vi "Commascript advanced.vi"() -> ()   [LabVIEW 2017]
panel:
  out "concatenated string":string
  out "stripped path":path
  out "appended path":path
  out "stripped path 2":path
  in  "Starting Pos":i16(slide)=128 scale=340.0..50.0
  in  "string":string
  out "new picture":picture
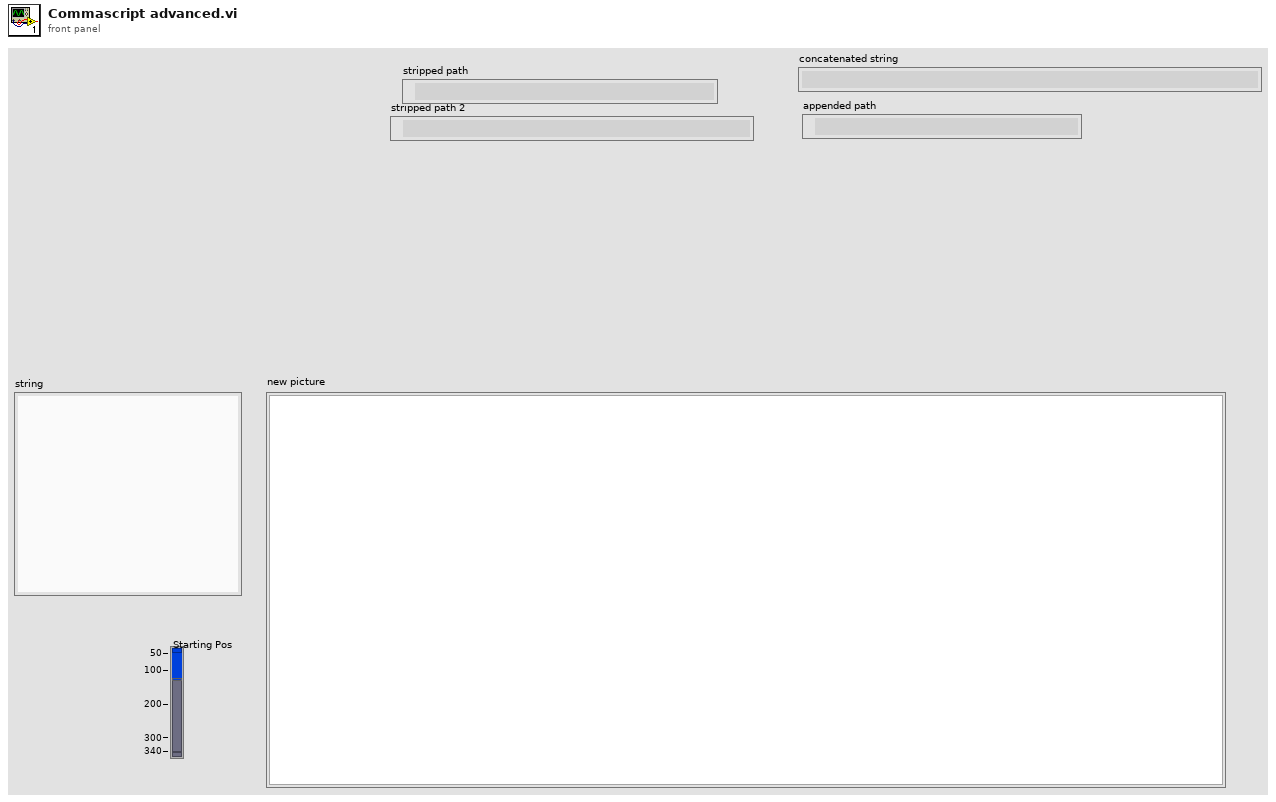
[diagram p1: front panel]
types:
  T1 = enum32{"invalid app kind", "Development System", "Run Time System", "Student Edition", "Embedded LabVIEW", "Evaluation", "Custom"}
  T2 = typedef "imagedata.ctl" = cluster{"image type":i32, "image depth":i32, "image":u8[], "mask":u8[], "colors":u32[], "Rectangle":cluster{"left":i16, "top":i16, "right":i16, "bottom":i16}}
  T3 = cluster{"Width":u16, "Style":enum32{"Solid", "Dash", "Dot", "DashDot", "DashDotDot"}}
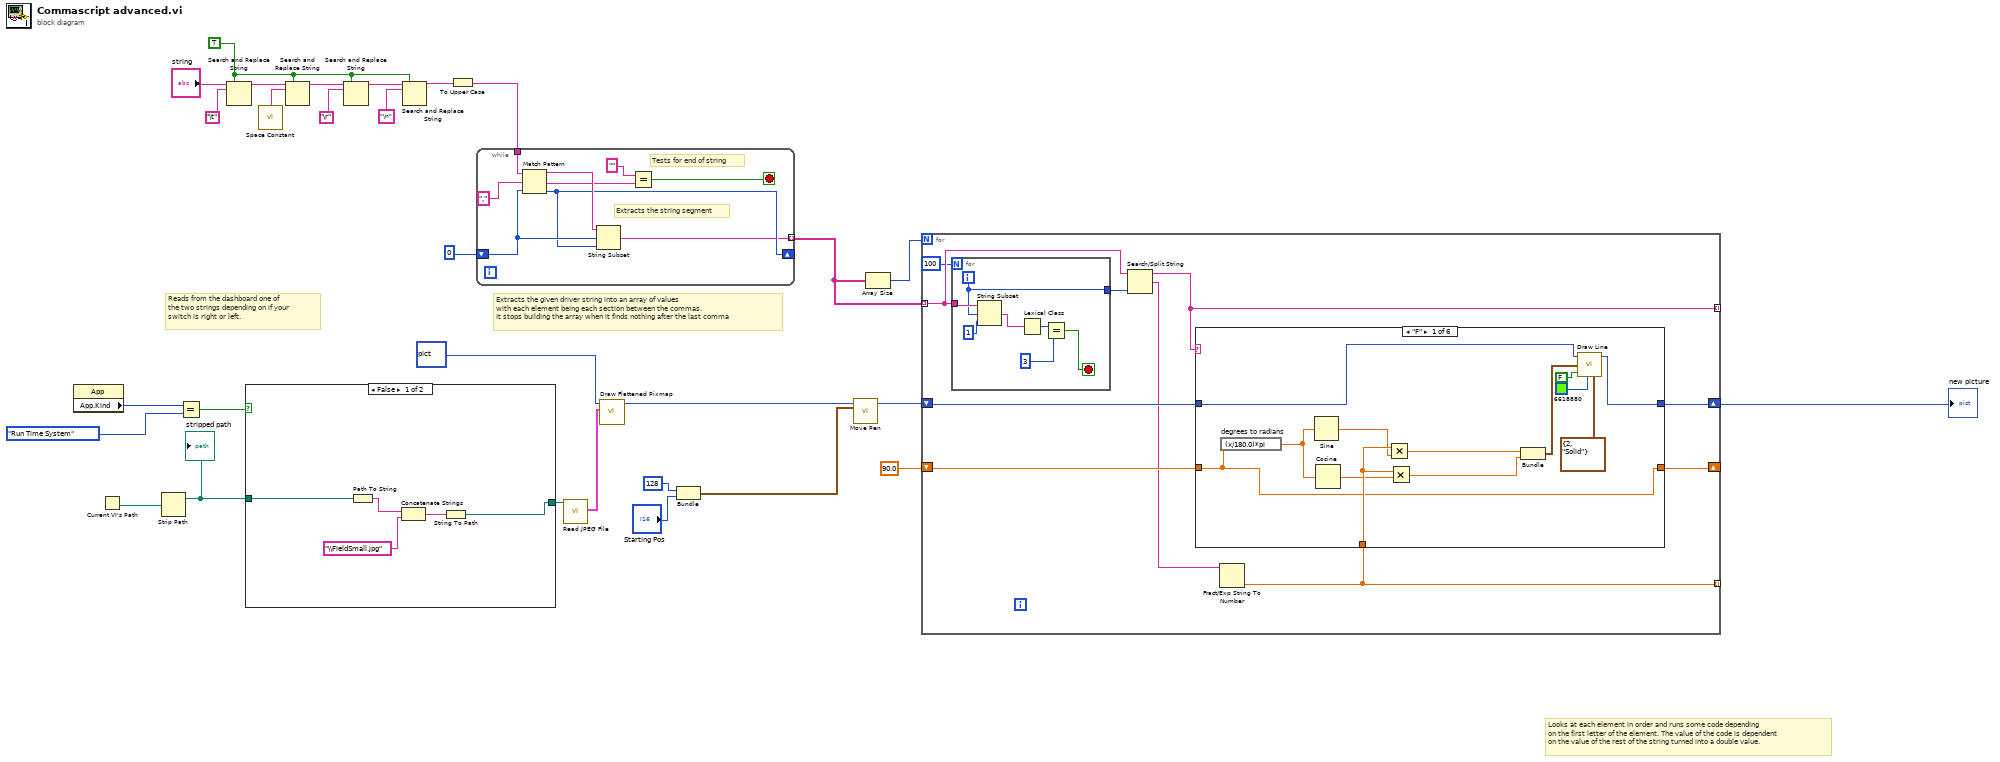
[diagram p0: block diagram]
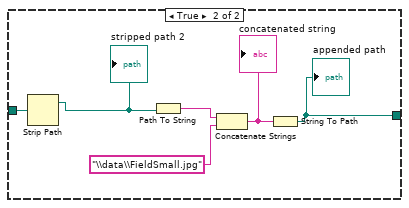
[diagram p2: hidden frame]
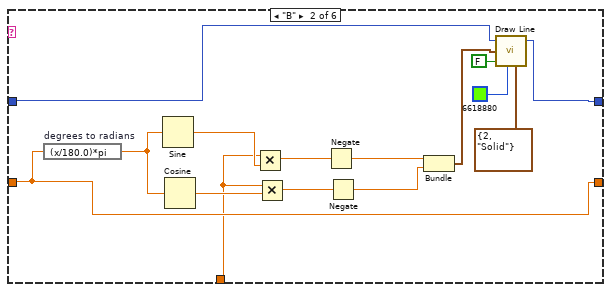
[diagram p3: hidden frame]
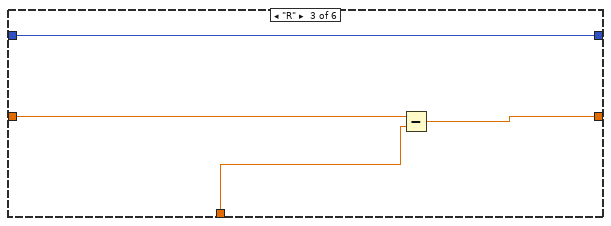
[diagram p4: hidden frame]
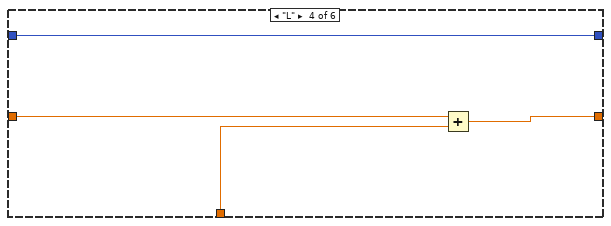
[diagram p5: hidden frame]
diagram:
  w11 = TRUE ("replace all? (F)")
  # "Reads from the dashboard one of\nthe two strings depending on if your\nswitch is right or left."
  # "Extracts the given driver string into an array of values \nwith each element being each section between the commas.\nIt stops building the array when it finds nothing after the last comma"
  # "Looks at each element in order and runs some code depending\non the first letter of the element. The value of the code is dependent\non the value of the rest of the string turned into a double value."
  n1 = property class="App"() -> ("App.Kind"=w5:T1)  [unwired: 2 in, 2 out]
  n2 = Current VI's Path() -> (path=w8:path)
  n3 = Strip Path(path=w8) -> (stripped path=w7:path)  [unwired: 1 out]
  "stripped path" <- w7
  n4 = Equal?(x=w5, y=T1."Run Time System") -> (x = y?=w3:bool)
  n5 = Search and Replace String(replace all?=w11, input string="string", search string="\t") -> (result string=w16:string)  [unwired: 5 in, 3 out]
  n6 = case shown="False" w3 {
    tunnel: w7 -> [w32 w40]
    tunnel: [w30 w35] -> w2
    frame False {
      n7 = Path To String(path=w32) -> (string=w31:string)
      n8 = Concatenate Strings(w31, "\\FieldSmall.jpg" ("name or relative path")) -> (w34:string)
      n9 = String To Path(string=w34) -> (path=w30:path)
    }
    frame True {
      n10 = Strip Path(path=w40) -> (stripped path=w39:path)  [unwired: 1 out]
      "stripped path 2" <- w39
      n11 = Path To String(path=w39) -> (string=w38:string)
      n12 = Concatenate Strings(w38, "\\data\\FieldSmall.jpg" ("name or relative path")) -> (w36:string)
      "concatenated string" <- w36
      n13 = String To Path(string=w36) -> (path=w35:path)
      "appended path" <- w35
    }
  }
  n14 = call <vilib>:"Space Constant.vi"() -> ("String"=w13:string)
  n15 = Search and Replace String(replace all?=w11, input string=w16, search string=w13) -> (result string=w17:string)  [unwired: 5 in, 3 out]
  n16 = Search and Replace String(replace all?=w11, input string=w17, search string="\r") -> (result string=w18:string)  [unwired: 5 in, 3 out]
  n17 = Search and Replace String(replace all?=w11, input string=w18, search string="\n") -> (result string=w10:string)  [unwired: 5 in, 3 out]
  n18 = To Upper Case(1:w10) -> (0:w9:string)
  n19 = while {
    shift-right: [w46] -> _
    shift-left: 0 ("offset past match") -> [w47]
    tunnel: [w45] -> w19 mode=indexing
    tunnel: w9 -> [w41]
    stop <- w42 stop-if-true
    # "Tests for end of string"
    # "Extracts the string segment"
    n20 = Match Pattern(string=w41, regular expression=",", offset (0)=w47) -> (before substring=w48:string, after substring=w44:string, offset past match=w46:i32)  [unwired: 1 out]
    n21 = String Subset(string=w48, offset (0)=w47, length (rest)=w46) -> (substring=w45:string)
    n22 = Equal?(x="", y=w44) -> (x = y?=w42:bool)
  }
  n23 = call <vilib>:"Read JPEG File.vi"("path to JPEG file"=w2) -> ("image data"=w1:T2)  [unwired: 8 in, 2 out]
  n24 = call <vilib>:"Draw Flattened Pixmap.vi"("image data"=w1, "picture"=picture data[5B]) -> ("new picture"=w24:picture)  [unwired: 7 in]
  n25 = Bundle("x"=i16 128, "Starting Pos"="Starting Pos") -> (w22:cluster{"x":i16, "Starting Pos":i16})  [unwired: 1 in]
  n26 = call <vilib>:"Move Pen.vi"("new position"=w22, "picture"=w24) -> ("new picture"=w28:picture)  [unwired: 3 in]
  n27 = Array Size(array=w19) -> (size(s)=w29:i32)
  n28 = for {
    N: w29 -> [_]
    tunnel: [w59] -> _ mode=indexing
    tunnel: [w52] -> _ mode=indexing
    tunnel: w19 -> [w53] mode=indexing
    shift-right: [w57] -> w26
    shift-left: w28 -> [w58]
    shift-right: [w55] -> _
    shift-left: 90.0 -> [w56]
    n29 = for {
      N: 100 -> [_]
      tunnel: w53 -> [w64]
      tunnel: [w61] -> w54
      i -> [w61]
      stop <- w60 stop-if-true
      n30 = String Subset(string=w64, offset (0)=w61, length (rest)=1 ("length (rest)")) -> (substring=w62:string)
      n31 = Lexical Class(1:w62) -> (0:w66:i16)
      n32 = Equal?(x=w66, y=i16 3) -> (x = y?=w60:bool)
    }
    n33 = Search/Split String(string=w53, offset (0)=w54) -> (substring before match=w52:string, match + rest of string=w51:string)  [unwired: 1 in, 1 out]
    n34 = Fract/Exp String To Number(string=w51) -> (number=w59:dbl)  [unwired: 3 in, 1 out]
    n35 = case shown="\"F\"" w52 {
      tunnel: w59 -> [w74 w86 w95 w99 _ _]
      tunnel: w58 -> [w78 w89 w98 w102 w104 w106]
      tunnel: [w77 w88 w98 w102 w104 w106] -> w57
      tunnel: w56 -> [w70 w87 w96 w100 w103 w105]
      tunnel: [w70 w87 w97 w101 w103 w105] -> w55
      frame "F" {
        n36 = expression code="(x/180.0)*pi" "degrees to radians"(w70) -> (w73:dbl)
        n37 = Sine(x=w73) -> (sin(x)=w71:dbl)
        n38 = Cosine(x=w73) -> (cos(x)=w72:dbl)
        n39 = Multiply(x=w74, y=w71) -> (x*y=w76:dbl)
        n40 = Multiply(x=w74, y=w72) -> (x*y=w75:dbl)
        n41 = Bundle(w76, w75) -> (w67:cluster{dbl, dbl})  [unwired: 1 in]
        n42 = call <vilib>:"Draw Line.vi"("picture"=w78, "end point"=w67, "absolute coordinates?(T)"=FALSE, "color(black)"=u32 6618880, "pen"=T3 {"Width"=2, "Style"=enum."Solid"}) -> ("new picture"=w77:picture)  [unwired: 4 in]
      }
      frame "B" {
        n43 = expression code="(x/180.0)*pi" "degrees to radians"(w87) -> (w92:dbl)
        n44 = Sine(x=w92) -> (sin(x)=w90:dbl)
        n45 = Cosine(x=w92) -> (cos(x)=w91:dbl)
        n46 = Multiply(x=w86, y=w90) -> (x*y=w85:dbl)
        n47 = Multiply(x=w86, y=w91) -> (x*y=w83:dbl)
        n48 = Negate(x=w85) -> (-x=w84:dbl)
        n49 = Negate(x=w83) -> (-x=w82:dbl)
        n50 = Bundle(w84, w82) -> (w93:cluster{dbl, dbl})  [unwired: 1 in]
        n51 = call <vilib>:"Draw Line.vi"("picture"=w89, "end point"=w93, "absolute coordinates?(T)"=FALSE, "color(black)"=u32 6618880, "pen"=T3 {"Width"=2, "Style"=enum."Solid"}) -> ("new picture"=w88:picture)  [unwired: 4 in]
      }
      frame "R" {
        n52 = Subtract(x=w96, y=w95) -> (x-y=w97:dbl)
      }
      frame "L" {
        n53 = Add(x=w100, y=w99) -> (x+y=w101:dbl)
      }
      frame "D", Default {
      }
      frame "IF" {
      }
    }
  }
  "new picture" <- w26
